vi "Stop Core.vi"(10 "final error code":i32, 11 "XBoxController-P in":refnum<class "XBoxController-P.lvclass">) -> (3 "XBoxController-P out":refnum<class "XBoxController-P.lvclass">)   [LabVIEW 2013, in "XBoxController-P.lvclass"]
doc: "(<B>Filename</B>: Actor Framework.lvlib:Actor.lvclass:Stop Core.vi)\n\nDefines what the actor does before it stops. Use the <B>final error code</B> input to determine whether the actor shut down in response to an error.\n\nBy default, this method does nothing. A descendant class may override it to define behavior, such as shutting down any processes the actor initiated in its override of the Actor Core method."
uses:
  XBoxController-P.lvclass
  Logical Systems/XBoxController/XBoxController.lvclass
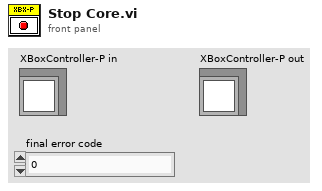
[diagram p1: front panel]
types:
  T1 = typedef "WPI_JoystickDevRef.ctl" = cluster{"Device":T2}
  T2 = typedef "WPI_JoystickDeviceEnum.ctl" = enum16{"USB 1", "USB 2", "USB 3", "USB 4", "Kinect 1", "Kinect 2"}
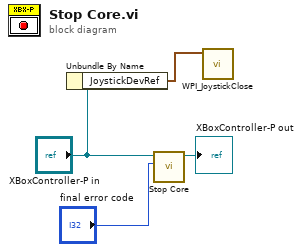
[diagram p0: block diagram]
diagram:
  n1 = Unbundle By Name("XBoxController-P in") -> ("JoystickDevRef"=w1:T1)
  n2 = call-parent "Stop Core.vi"("final error code"="final error code", "Actor in"="XBoxController-P in") -> ("Actor out"=→"XBoxController-P out":refnum<class "XBoxController-P.lvclass">)  [unwired: 9 in]
  n3 = call <vilib>:"WPI_JoystickClose.vi"("JoystickDevRef"=w1) -> ()  [unwired: 11 in]
